vi "Autonomous Independent.vi"() -> ()   [LabVIEW 2016]
doc: "This VI is called when autonomous begins, and will automatically be terminated when autonomous ends. You can carry out timed or sensor driven robot movement independently without needing to return to the caller."
uses:
  <vilib>/Rock Robotics/WPI/SafetyOutput/WPI_SafetyOutputConfigMenu.ctl
  <vilib>/Rock Robotics/WPI/Utilities/WPI_GetSetVariantRefNum.vi
  <vilib>/Rock Robotics/Network Tables/NT Read String.vi
  <vilib>/Rock Robotics/WPI/Ultrasonic/WPI_SonarMB1010AnalogRefNum Registry Get.vi
  <vilib>/Rock Robotics/Network Tables/NT Read Number.vi
  <vilib>/Rock Robotics/WPI/Ultrasonic/WPI_SonarMB1010AnalogGetRange.vi
  <vilib>/Rock Robotics/WPI/RobotDrive/WPI_RobotDriveArcadeDrive_Standard(NoSaturation).vi
  <vilib>/Rock Robotics/Network Tables/NT Write Numeric Array.vi
panel:
  in  "Angle to Lift":dbl
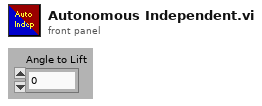
[diagram p1: front panel]
types:
  T1 = typedef "WPI_JoystickDevRef.ctl" = cluster{"Device":T2}
  T2 = typedef "WPI_JoystickDeviceEnum.ctl" = enum16{"USB 0", "USB 1", "USB 2", "USB 3", "USB 4", "USB 5"}
  T3 = typedef "WPI_SafetyOutputConfigMenu.ctl" = enum16{"Enable", "Disable"}
  T4 = typedef "WPI_SonarMB1010AnalogDeviceRef.ctl" = cluster{"AIDeviceRef":T5, "Scaling factor (V/in)":dbl, "Average Bits":u8}
  T5 = typedef "WPI_AnalogChannelDevRef.ctl" = cluster{"DevStatus":errorcluster, "Analog Channel":T6}
  T6 = typedef "FPGA_AIChannel.ctl" = enum8{"AI 0", "AI 1", "AI 2", "AI 3", "AI MXP 0", "AI MXP 1", "AI MXP 2", "AI MXP 3", "Invalid"}
  T7 = typedef "WPI_RobotDriveDevRef.ctl" = cluster{"DevStatus":errorcluster, "Motors[]":T8[], "Square Inputs":bool, "Max Output":dbl}
  T8 = typedef "WPI_MotorControlDeviceRef.ctl" = cluster{"DeviceStatus":errorcluster, "Type":T9, "PWM":cluster{"PWM Channel":T10, "DeadBand":T11}, "CAN":cluster{"Device Number":u8, "SetOutput VI Ref":variant, "GetOutput VI Ref":variant, "Enable VI Ref":variant, "Disable VI Ref":variant, "Data":variant}, "Invert":bool}
  T9 = typedef "WPI_MotorControlType.ctl" = enum16{"PWM", "CAN"}
  T10 = typedef "FPGA_DIOPWMChannel.ctl" = enum8{"PWM 0", "PWM 1", "PWM 2", "PWM 3", "PWM 4", "PWM 5", "PWM 6", "PWM 7", "PWM 8", "PWM 9", "PWM MXP 0", "PWM MXP 1", "PWM MXP 2", "PWM MXP 3", "PWM MXP 4", "PWM MXP 5", "PWM MXP 6", "PWM MXP 7", "PWM MXP 8", "PWM MXP 9", "Invalid"}
  T11 = typedef "WPI_PWMDeadband.ctl" = cluster{"Name":string, "maxPositivePwm":i32, "minPositivePwm":i32, "centerPwm":i32, "maxNegativePwm":i32, "minNegativePwm":i32, "angularRange":u16}
  T12 = typedef "WPI_GyroDevRef.ctl" = cluster{"DevStatus":errorcluster, "Analog Channel":T6, "Offset":dbl, "Gain (VoltsPerDegree/Second)":dbl, "Gyro Type":enum16{"Analog", "XRS450"}, "Handle":i32, "SPI Bus":T13, "Device Found":bool, "Sample Rate":dbl, "Calibrate On Open":bool}
  T13 = typedef "spi_bus.ctl" = enum16{"SPI On-Board, CS0", "SPI On-Board, CS1", "SPI On-Board, CS2", "SPI On-Board, CS3", "SPI MXP", "Invalid"}
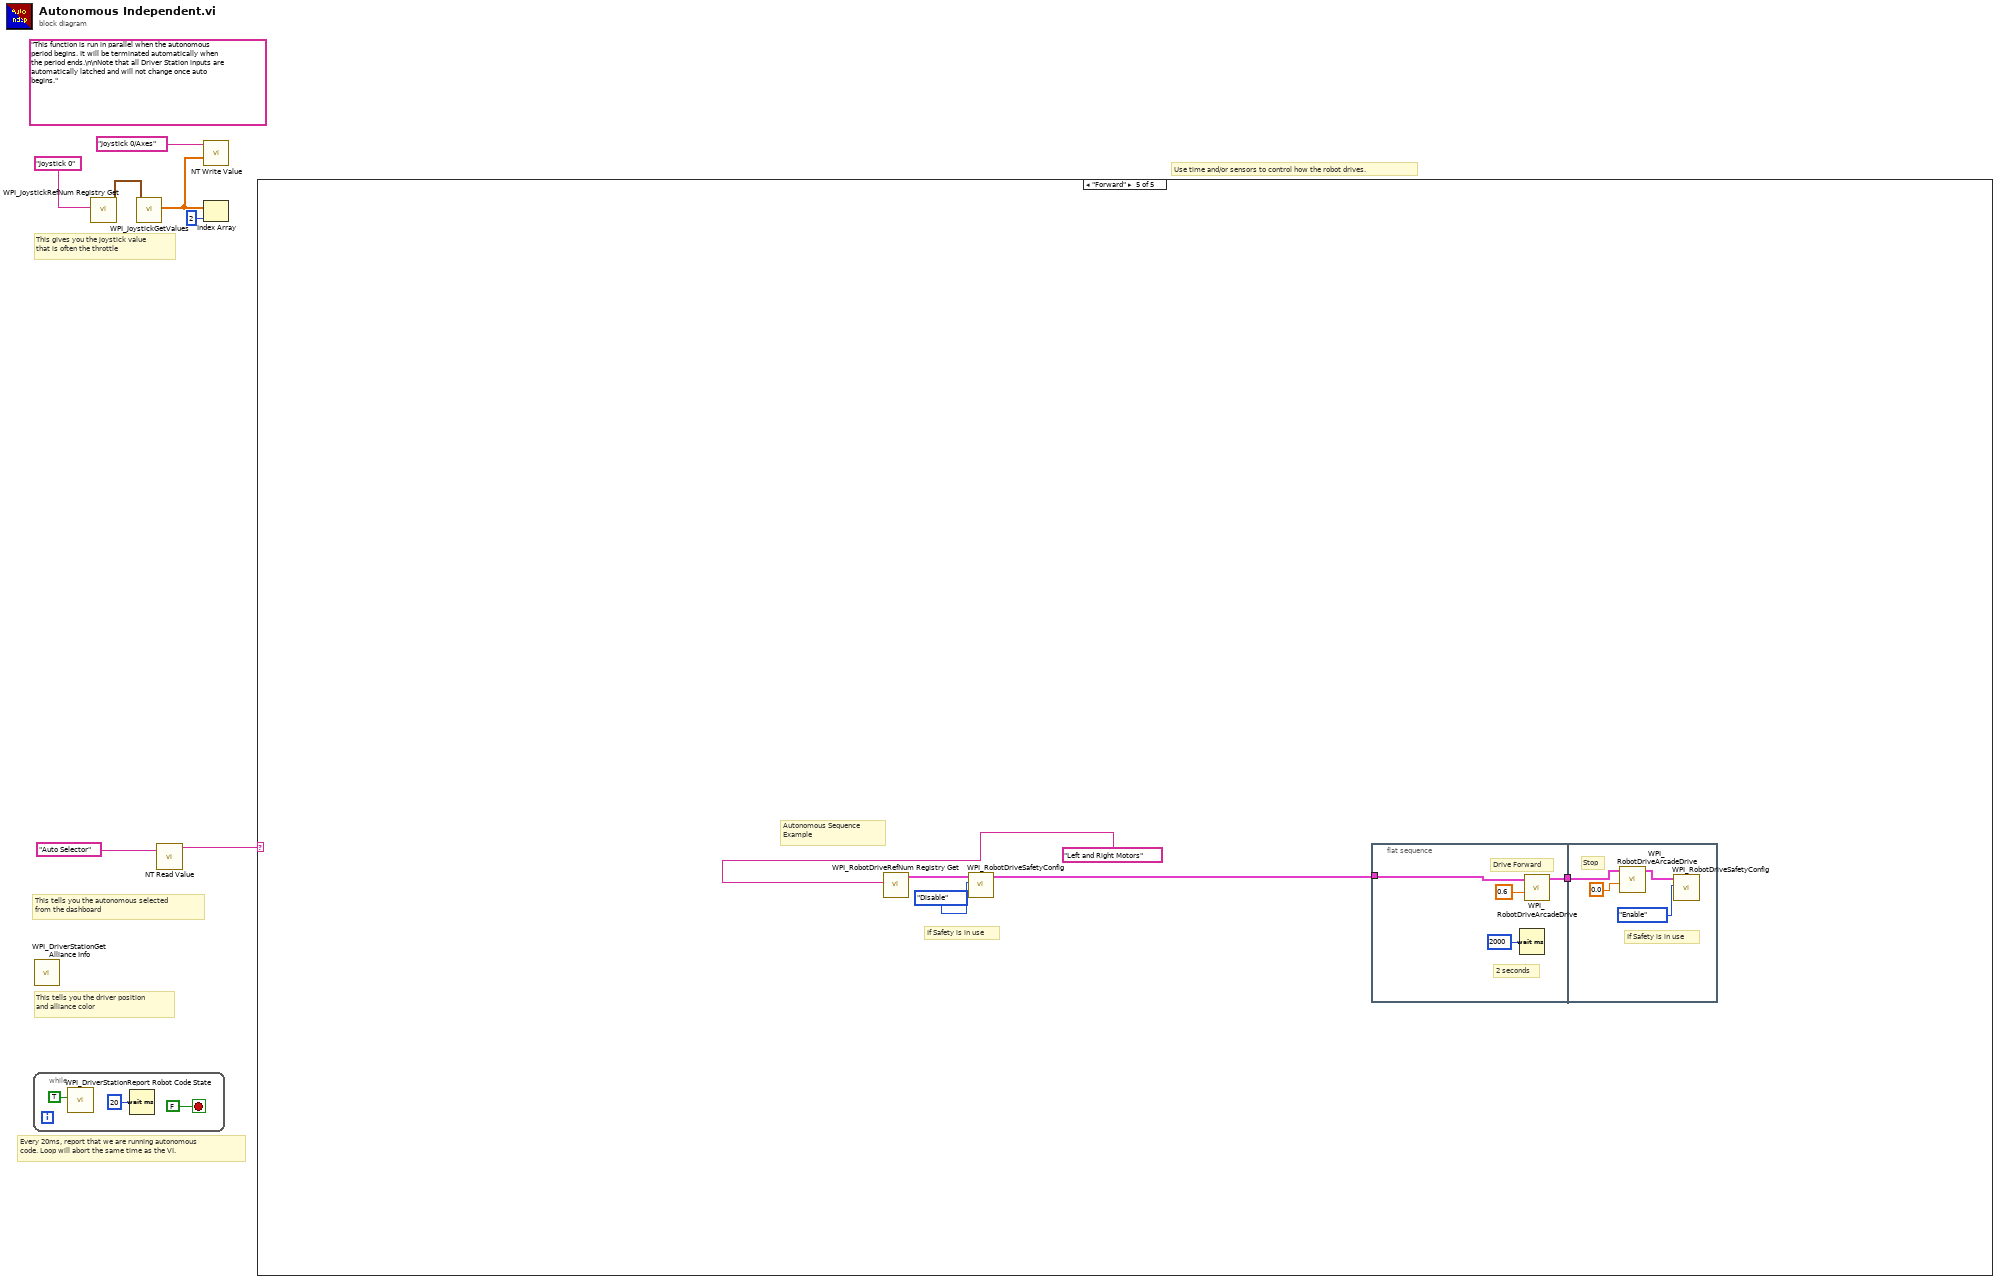
[diagram p0: block diagram]
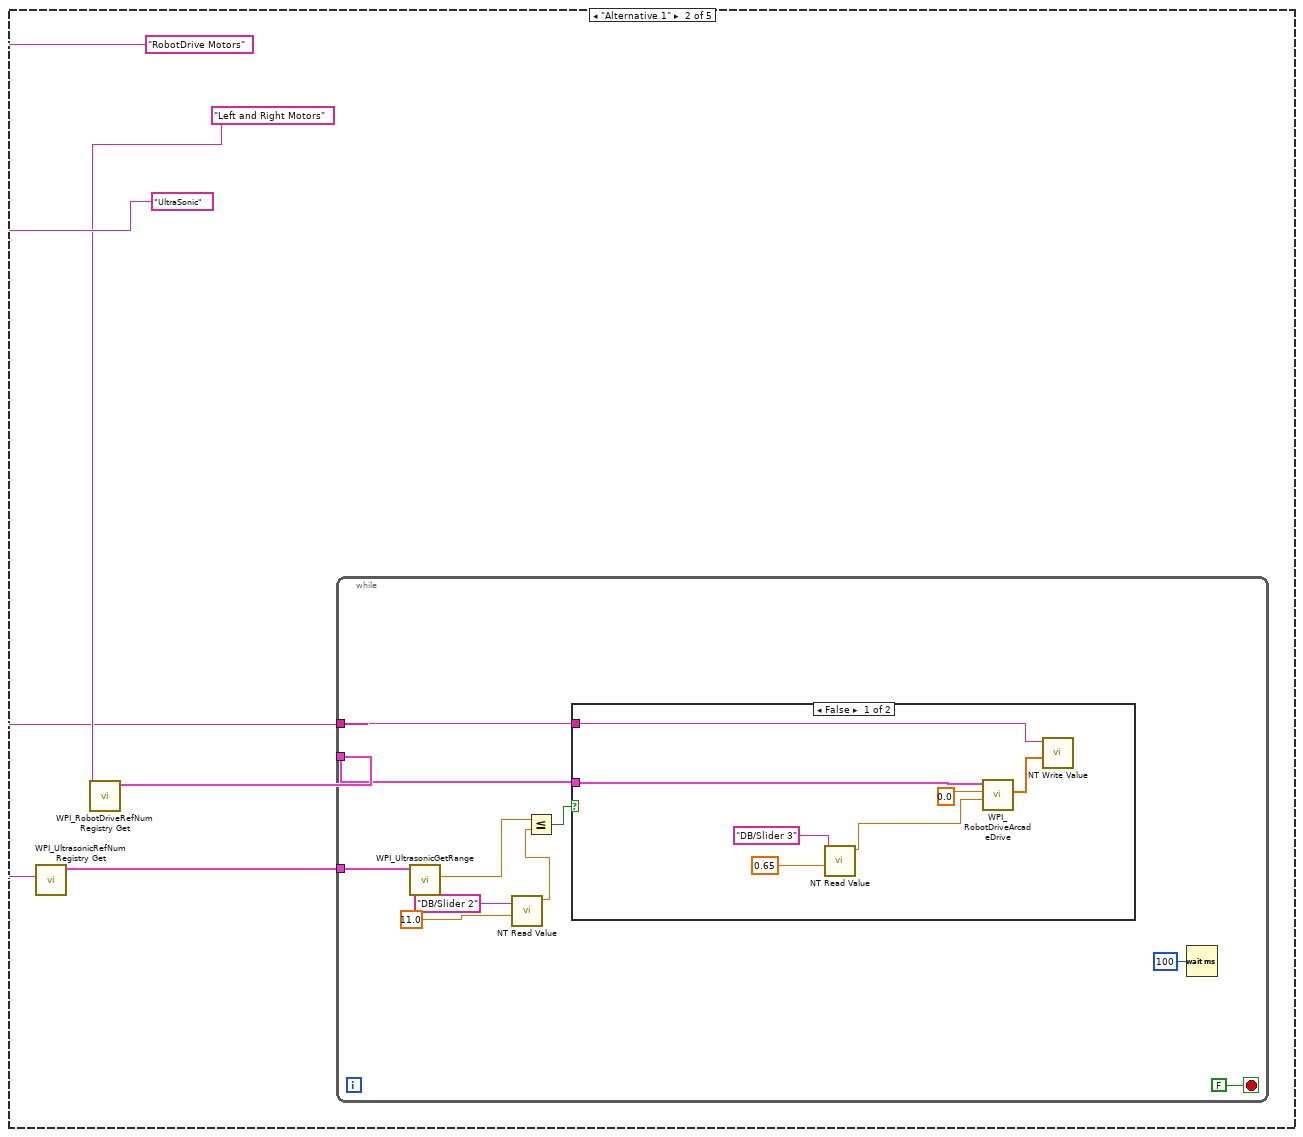
[diagram p3: hidden frame]
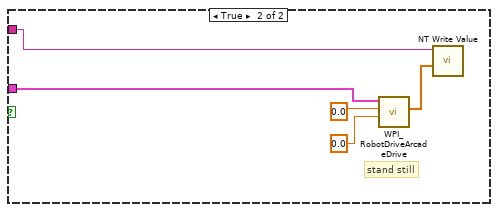
[diagram p4: hidden frame]
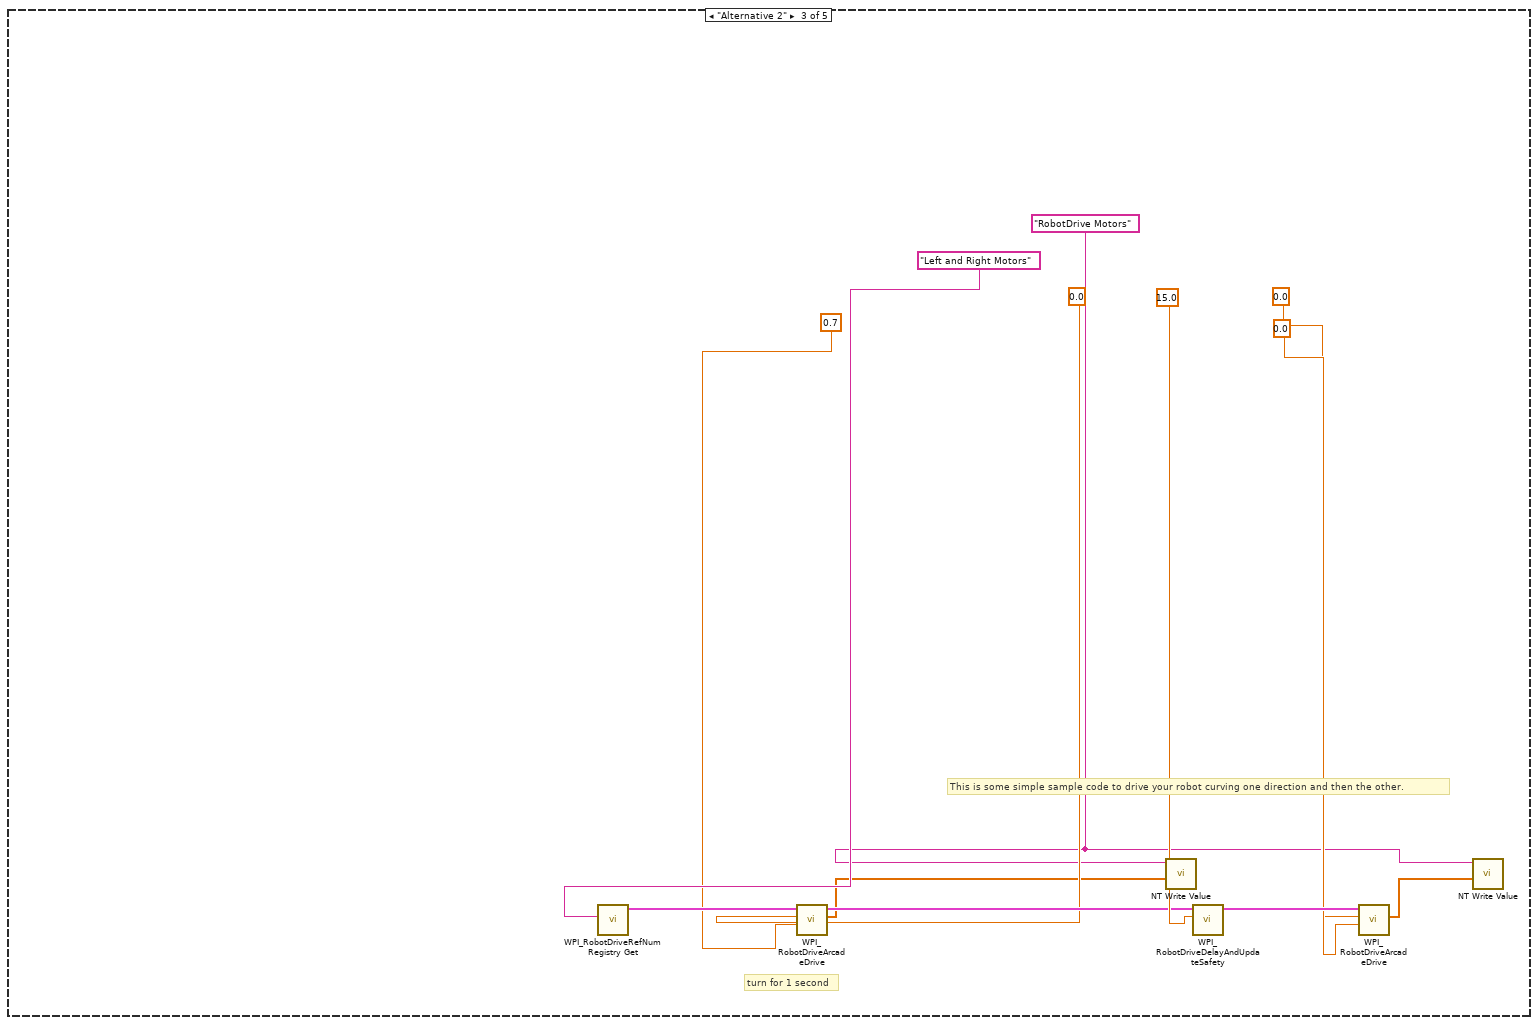
[diagram p5: hidden frame]
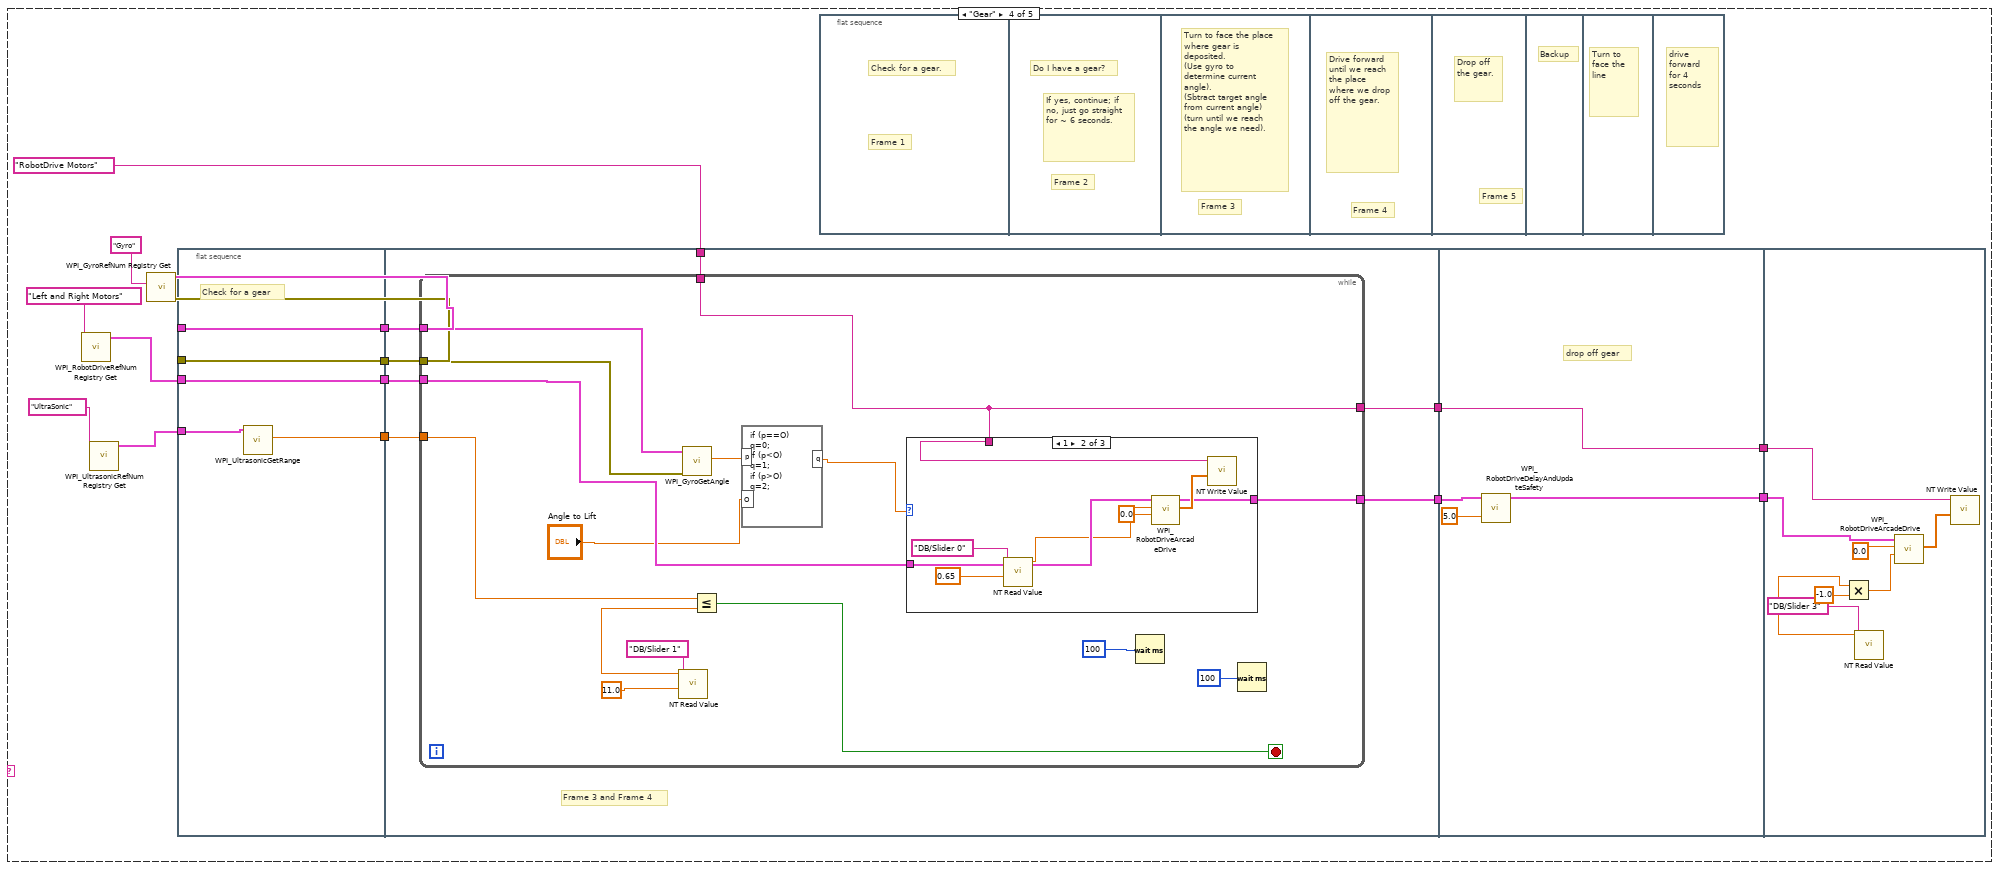
[diagram p6: hidden frame]
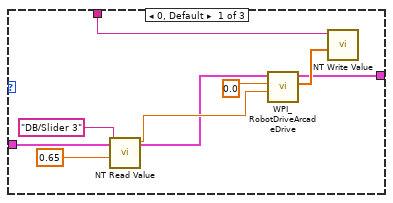
[diagram p7: hidden frame]
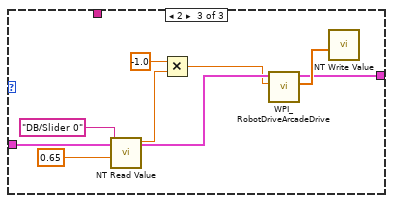
[diagram p8: hidden frame]
diagram:
  (unwired) "This function is run in parallel when the autonomous period begins. It will be terminated automatically when the period ends.\n\nNote that all Driver Station inputs are automatically latched and will not change once auto begins."
  # "This tells you the autonomous selected\nfrom the dashboard"
  # "Every 20ms, report that we are running autonomous\ncode. Loop will abort the same time as the VI."
  # "This gives you the joystick value\nthat is often the throttle"
  # "Use time and/or sensors to control how the robot drives."
  # "This tells you the driver position\nand alliance color"
  n1 = while {
    stop <- FALSE stop-if-true
    n2 = call <vilib>:"WPI_DriverStationReport Robot Code State.vi"("Autonomous"=TRUE) -> ()  [unwired: 10 in, 1 out]
    n3 = Wait (ms)(milliseconds to wait=u32 20) -> ()  [unwired: 1 out]
  }
  n4 = call <vilib>:"WPI_DriverStationGet Alliance Info.vi"() -> ()  [unwired: 12 out]
  n5 = call <vilib>:"WPI_JoystickRefNum Registry Get.vi"("refnum name"="Joystick 0") -> ("JoystickDevRef"=w6:T1)  [unwired: 1 in, 9 out]
  n6 = call <vilib>:"WPI_JoystickGetValues.vi"("JoystickDevRef"=w6) -> ("Axes"=w2:dbl[])  [unwired: 6 in, 4 out]
  n7 = call-poly <vilib>:"NT Read Value.vi"("Name"="Auto Selector") -> ("String"=w3:string)  [unwired: 9 in, 1 out]
  n8 = call-poly <vilib>:"NT Write Value.vi"("Numeric Array"=w2, "Name"="Joystick 0/Axes") -> ()  [unwired: 9 in, 1 out]
  n9 = Index Array(array=w2, index=2) -> ()  [unwired: 1 out]
  n10 = case shown="\"Forward\"" w3 {
    frame Default {
      # "You can put your main auto here, or you can right-click on the case and make any\nother frame be the default case."
      # "This is the frame that will execute if no selection is made, or if it is not recognized"
    }
    frame "Alternative 1" {
      n11 = call-poly <vilib>:"WPI_UltrasonicRefNum Registry Get.vi"("refnum name"="UltraSonic") -> ("SonarMB1010AnalogDevRef"=w11:T4)  [unwired: 9 in, 1 out]
      n12 = call <vilib>:"WPI_RobotDriveRefNum Registry Get.vi"("refnum name"="Left and Right Motors") -> ("RobotDriveDevRef"=w12:T7)  [unwired: 1 in, 9 out]
      n13 = while {
        tunnel: "RobotDrive Motors" ("Name") -> [w24]
        tunnel: w12 -> [w23]
        tunnel: w11 -> [w21]
        stop <- FALSE stop-if-true
        n14 = call-poly <vilib>:"WPI_UltrasonicGetRange.vi"("SonarMB1010AnalogDevRef"=w21) -> ("Distance"=w22:dbl)  [unwired: 8 in, 2 out]
        n15 = call-poly <vilib>:"NT Read Value.vi"("Default Value"=11.0 ("y"), "Name"="DB/Slider 2") -> ("Numeric"=w18:dbl)  [unwired: 8 in, 1 out]
        n16 = Less Or Equal?(x=w22, y=w18) -> (x <= y?=w25:bool)
        n17 = case shown="False" w25 {
          tunnel: w24 -> [w27 w33]
          tunnel: w23 -> [w26 w34]
          frame False {
            n18 = call-poly <vilib>:"NT Read Value.vi"("Default Value"=0.65, "Name"="DB/Slider 3") -> ("Numeric"=w30:dbl)  [unwired: 8 in, 1 out]
            n19 = call-poly <vilib>:"WPI_RobotDriveArcadeDrive.vi"("Y axis value"=w30, "X axis value"=0.0, "RobotDriveDevRef"=w26) -> ("Motor Values"=w29:dbl[])  [unwired: 1 in, 7 out]
            n20 = call-poly <vilib>:"NT Write Value.vi"("Numeric Array"=w29, "Name"=w27) -> ()  [unwired: 9 in, 1 out]
          }
          frame True {
            # "stand still"
            n21 = call-poly <vilib>:"WPI_RobotDriveArcadeDrive.vi"("Y axis value"=0.0 ("X axis value"), "X axis value"=0.0, "RobotDriveDevRef"=w34) -> ("Motor Values"=w37:dbl[])  [unwired: 1 in, 7 out]
            n22 = call-poly <vilib>:"NT Write Value.vi"("Numeric Array"=w37, "Name"=w33) -> ()  [unwired: 9 in, 1 out]
          }
        }
        n23 = Wait (ms)(milliseconds to wait=u32 100) -> ()  [unwired: 1 out]
      }
    }
    frame "Alternative 2" {
      w40 = "RobotDrive Motors" ("Name")
      # "This is some simple sample code to drive your robot curving one direction and then the other."
      # "turn for 1 second"
      n24 = call <vilib>:"WPI_RobotDriveRefNum Registry Get.vi"("refnum name"="Left and Right Motors") -> ("RobotDriveDevRef"=w49:T7)  [unwired: 1 in, 9 out]
      n25 = call-poly <vilib>:"WPI_RobotDriveArcadeDrive.vi"("Y axis value"=0.7 ("Default Value"), "X axis value"=0.0, "RobotDriveDevRef"=w49) -> ("Motor Values"=w39:dbl[], "RobotDriveDevRef"=w45:T7)  [unwired: 1 in, 6 out]
      n26 = call-poly <vilib>:"NT Write Value.vi"("Numeric Array"=w39, "Name"=w40) -> ()  [unwired: 9 in, 1 out]
      n27 = call <vilib>:"WPI_RobotDriveDelayAndUpdateSafety.vi"("Delay (s)"=15.0, "RobotDriveDevRef"=w45) -> ("RobotDriveDevRef 2"=w46:T7)  [unwired: 8 in, 1 out]
      n28 = call-poly <vilib>:"WPI_RobotDriveArcadeDrive.vi"("Y axis value"=0.0 ("X axis value"), "X axis value"=0.0, "RobotDriveDevRef"=w46) -> ("Motor Values"=w41:dbl[])  [unwired: 1 in, 7 out]
      n29 = call-poly <vilib>:"NT Write Value.vi"("Numeric Array"=w41, "Name"=w40) -> ()  [unwired: 9 in, 1 out]
    }
    frame "Gear" {
      n30 = call <vilib>:"WPI_RobotDriveRefNum Registry Get.vi"("refnum name"="Left and Right Motors") -> ("RobotDriveDevRef"=w60:T7)  [unwired: 1 in, 9 out]
      n31 = call-poly <vilib>:"WPI_UltrasonicRefNum Registry Get.vi"("refnum name"="UltraSonic") -> ("SonarMB1010AnalogDevRef"=w57:T4)  [unwired: 9 in, 1 out]
      n32 = call <vilib>:"WPI_GyroRefNum Registry Get.vi"("refnum name"="Gyro") -> ("error out"=w55:errorcluster, "GyroDevRef"=w64:T12)  [unwired: 9 in]
      n33 = flat-sequence {
        tunnel: w64 -> [w70]
        tunnel: [w70] -> w63
        tunnel: [w69] -> w61
        tunnel: w60 -> [w69]
        tunnel: w57 -> [w68]
        tunnel: [w67] -> w56
        tunnel: w55 -> [w67]
        tunnel: [w66] -> w54
        tunnel: w63 -> [w77]
        tunnel: w61 -> [w76]
        tunnel: "RobotDrive Motors" ("Name") -> [w75]
        tunnel: w56 -> [w74]
        tunnel: w54 -> [w73]
        tunnel: [w72] -> w53
        tunnel: [w71] -> w52
        tunnel: w53 -> [w120]
        tunnel: w52 -> [w119]
        tunnel: [w119] -> w51
        tunnel: [w118] -> w50
        tunnel: w51 -> [w125]
        tunnel: w50 -> [w124]
        frame #0 {
          # "Check for a gear"
          n34 = call-poly <vilib>:"WPI_UltrasonicGetRange.vi"("SonarMB1010AnalogDevRef"=w68) -> ("Distance"=w66:dbl)  [unwired: 8 in, 2 out]
        }
        frame #1 {
          # "Frame 3 and Frame 4"
          n35 = while {
            tunnel: w77 -> [w91]
            tunnel: w76 -> [w90]
            tunnel: w75 -> [w79]
            tunnel: w74 -> [w89]
            tunnel: w73 -> [w82]
            tunnel: [w80] -> w72
            tunnel: [w79] -> w71
            stop <- w81 stop-if-true
            n36 = call-poly <vilib>:"NT Read Value.vi"("Default Value"=11.0 ("y"), "Name"="DB/Slider 1") -> ("Numeric"=w83:dbl)  [unwired: 8 in, 1 out]
            n37 = call <vilib>:"WPI_GyroGetAngle.vi"("error in"=w89, "GyroDevRef"=w91) -> ("Angle"=w87:dbl)  [unwired: 5 in, 4 out]
            n38 = Less Or Equal?(x=w82, y=w83) -> (x <= y?=w81:bool)
            n39 = formula code="if (p==O)\nq=0;\nif (p<O)\nq=1;\nif (p>O)\nq=2;"("p"=w87, "O"="Angle to Lift") -> ("q"=w86:dbl)
            n40 = case shown="1" w86 {
              tunnel: w90 -> [w95 w105 w113]
              tunnel: w79 -> [w94 w104 _]
              tunnel: [w93 w101 w109] -> w80
              frame 0, Default {
                n41 = call-poly <vilib>:"NT Read Value.vi"("Default Value"=0.65, "Name"="DB/Slider 3") -> ("Numeric"=w98:dbl)  [unwired: 8 in, 1 out]
                n42 = call-poly <vilib>:"WPI_RobotDriveArcadeDrive.vi"("Y axis value"=w98, "X axis value"=0.0, "RobotDriveDevRef"=w95) -> ("Motor Values"=w97:dbl[], "RobotDriveDevRef"=w93:T7)  [unwired: 1 in, 6 out]
                n43 = call-poly <vilib>:"NT Write Value.vi"("Numeric Array"=w97, "Name"=w94) -> ()  [unwired: 9 in, 1 out]
              }
              frame 1 {
                n44 = call-poly <vilib>:"NT Read Value.vi"("Default Value"=0.65, "Name"="DB/Slider 0") -> ("Numeric"=w103:dbl)  [unwired: 8 in, 1 out]
                n45 = call-poly <vilib>:"WPI_RobotDriveArcadeDrive.vi"("Y axis value"=0.0, "X axis value"=w103, "RobotDriveDevRef"=w105) -> ("Motor Values"=w106:dbl[], "RobotDriveDevRef"=w101:T7)  [unwired: 1 in, 6 out]
                n46 = call-poly <vilib>:"NT Write Value.vi"("Numeric Array"=w106, "Name"=w104) -> ()  [unwired: 9 in, 1 out]
              }
              frame 2 {
                n47 = call-poly <vilib>:"NT Read Value.vi"("Default Value"=0.65, "Name"="DB/Slider 0") -> ("Numeric"=w112:dbl)  [unwired: 8 in, 1 out]
                n48 = Multiply(x=-1.0, y=w112) -> (x*y=w111:dbl)
                n49 = call-poly <vilib>:"WPI_RobotDriveArcadeDrive.vi"("X axis value"=w111, "RobotDriveDevRef"=w113) -> ("Motor Values"=w116:dbl[], "RobotDriveDevRef"=w109:T7)  [unwired: 2 in, 6 out]
                n50 = call-poly <vilib>:"NT Write Value.vi"("Numeric Array"=w116) -> ()  [unwired: 10 in, 1 out]
              }
            }
            n51 = Wait (ms)(milliseconds to wait=u32 100) -> ()  [unwired: 1 out]
          }
          n52 = Wait (ms)(milliseconds to wait=u32 100) -> ()  [unwired: 1 out]
        }
        frame #2 {
          # "drop off gear"
          n53 = call <vilib>:"WPI_RobotDriveDelayAndUpdateSafety.vi"("Delay (s)"=5.0, "RobotDriveDevRef"=w120) -> ("RobotDriveDevRef 2"=w118:T7)  [unwired: 8 in, 1 out]
        }
        frame #3 {
          n54 = call-poly <vilib>:"NT Read Value.vi"("Name"="DB/Slider 3") -> ("Numeric"=w123:dbl)  [unwired: 9 in, 1 out]
          n55 = Multiply(x=w123, y=-1.0) -> (x*y=w121:dbl)
          n56 = call-poly <vilib>:"WPI_RobotDriveArcadeDrive.vi"("Y axis value"=w121, "X axis value"=0.0, "RobotDriveDevRef"=w124) -> ("Motor Values"=w127:dbl[])  [unwired: 1 in, 7 out]
          n57 = call-poly <vilib>:"NT Write Value.vi"("Numeric Array"=w127, "Name"=w125) -> ()  [unwired: 9 in, 1 out]
        }
      }
      n58 = flat-sequence {
        frame #0 {
          # "Frame 1"
          # "Check for a gear."
        }
        frame #1 {
          # "Frame 2"
          # "If yes, continue; if no, just go straight for ~ 6 seconds."
          # "Do I have a gear?"
        }
        frame #2 {
          # "Frame 3"
          # "Turn to face the place where gear is deposited.\n(Use gyro to determine current angle).\n(Sbtract target angle from current angle)\n(turn until we reach the angle we need)."
        }
        frame #3 {
          # "Frame 4"
          # "Drive forward until we reach the place where we drop off the gear."
        }
        frame #4 {
          # "Frame 5"
          # "Drop off the gear."
        }
        frame #5 {
          # "Backup"
        }
        frame #6 {
          # "Turn to face the line"
        }
        frame #7 {
          # "drive forward for 4 seconds"
        }
      }
    }
    frame "Forward" {
      # "If Safety is in use"
      # "Autonomous Sequence\nExample"
      n59 = call <vilib>:"WPI_RobotDriveRefNum Registry Get.vi"("refnum name"="Left and Right Motors") -> ("RobotDriveDevRef"=w132:T7)  [unwired: 9 in, 1 out]
      n60 = call <vilib>:"WPI_RobotDriveSafetyConfig.vi"("mode"=WPI_SafetyOutputConfigMenu."Disable", "RobotDriveDevRef"=w132) -> ("RobotDriveDevRef"=w131:T7)  [unwired: 8 in, 1 out]
      n61 = flat-sequence {
        tunnel: w131 -> [w135]
        tunnel: [w134] -> w129
        tunnel: w129 -> [w138]
        frame #0 {
          # "2 seconds"
          # "Drive Forward"
          n62 = Wait (ms)(milliseconds to wait=u32 2000) -> ()  [unwired: 1 out]
          n63 = call-poly <vilib>:"WPI_RobotDriveArcadeDrive.vi"("Y axis value"=0.6 ("Left axis value"), "RobotDriveDevRef"=w135) -> ("RobotDriveDevRef"=w134:T7)  [unwired: 7 in, 2 out]
        }
        frame #1 {
          # "If Safety is in use"
          # "Stop"
          n64 = call-poly <vilib>:"WPI_RobotDriveArcadeDrive.vi"("Y axis value"=0.0 ("Left axis value"), "RobotDriveDevRef"=w138) -> ("RobotDriveDevRef"=w139:T7)  [unwired: 7 in, 2 out]
          n65 = call <vilib>:"WPI_RobotDriveSafetyConfig.vi"("mode"=WPI_SafetyOutputConfigMenu."Enable", "RobotDriveDevRef"=w139) -> ()  [unwired: 8 in, 2 out]
        }
      }
    }
  }
